vi "Define 1D Heat PDE BC (VIRef).vi"(0 "PDE in":refnum<class "NI_PDE.lvclass">, 1 "data":variant, 5 "Boundary Condition":refnum<vi>, 7 "type":T2 items=["Dirichlet", "Neumann"], 9 "position":T1 items=["Start X", "End X"], 11 "error in (no error)":errorcluster) -> (4 "PDE out":refnum<class "NI_PDE.lvclass">, 15 "error out":errorcluster)   [LabVIEW 2017, in "NI_PDE.lvlib"]
doc: "Defines the boundary condition of partial differential equations. You must manually select the polymorphic instance to use."
uses:
  <vilib>/gmath/NI_PDE.lvlib
  <vilib>/gmath/pde.llb/Common/PDE_BC Type.ctl
  <vilib>/gmath/pde.llb/PDEClass/NI_PDE.lvclass
  <vilib>/gmath/pde.llb/Common/PDE_BC Position 1D.ctl
  <vilib>/gmath/pde.llb/BCClass/BC_Evolut_1D_VIRef/NI_BC_Evolut_1D_VIRef.lvclass
  e:/builds/penguin/labview/branches/2017/dev/dist/vi.lib/gmath/pde.llb/BCClass/NI_BC.lvclass
  <vilib>/gmath/pde.llb/PDEClass/PDE_Heat_1D/NI_PDE_Heat_1D.lvclass
  e:/builds/penguin/labview/branches/2017/dev/dist/vi.lib/gmath/pde.llb/PDEClass/NI_PDE.lvclass
  <vilib>/gmath/pde.llb/BCClass/BC_Evolut_1D_VIRef/BC Data.ctl
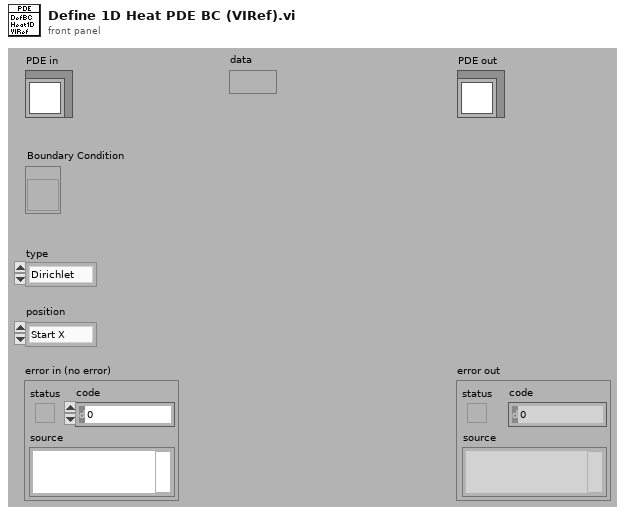
[diagram p1: front panel]
types:
  T1 = typedef "NI_PDE.lvlib/PDE_BC Position 1D.ctl" = i32
  T2 = typedef "NI_PDE.lvlib/PDE_BC Type.ctl" = i32
  T3 = typedef "NI_PDE.lvlib/NI_BC_Evolut_1D_VIRef.lvclass/BC Data.ctl" = cluster{"type":T2, "position":T1, "G":refnum<vi>, "data":variant}
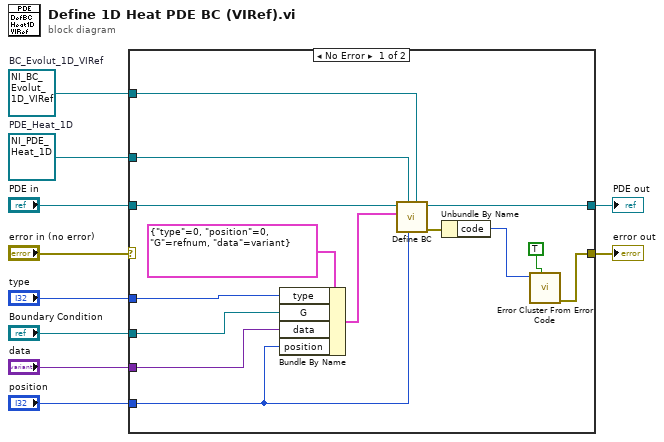
[diagram p0: block diagram]
diagram:
  w2 = refnum<class "NI_PDE_Heat_1D.lvclass"> refnum  # PDE_Heat_1D
  w1 = refnum<class "NI_BC_Evolut_1D_VIRef.lvclass"> refnum  # BC_Evolut_1D_VIRef
  n1 = case shown="No Error" "error in (no error)" {
    selector: "error in (no error)" -> [_ w26]
    tunnel: "PDE in" -> [w13 w25]
    tunnel: [w21 w25] -> w9
    tunnel: "position" -> [w15 _]
    tunnel: "data" -> [w16 _]
    tunnel: "Boundary Condition" -> [w17 _]
    tunnel: "type" -> [w18 _]
    tunnel: [w22 w26] -> w4
    tunnel: w2 -> [w12 _]
    tunnel: w1 -> [w11 _]
    frame No Error {
      n2 = Bundle By Name(cluster=T3 {"type"=0, "position"=0, "G"=refnum, "data"=variant} ("BC data"), "type"=w18, "G"=w17, "data"=w16, "position"=w15) -> (w14:T3)
      n3 = call <vilib>:"Define BC.vi"("target BC"=w11, "index"=w15, "target PDE"=w12, "BC"=w14, "PDE in"=w13) -> ("error out"=w20:errorcluster, "PDE out"=w21:refnum<class "NI_PDE.lvclass">)  [unwired: 2 in, 3 out]
      n4 = Unbundle By Name(w20) -> ("code"=w24:i32)
      n5 = call <vilib>:"Error Cluster From Error Code.vi"("show call chain? (False)"=TRUE, "error code (0)"=w24) -> ("error out"=w22:errorcluster)  [unwired: 1 in, 6 out]
    }
    frame Error {
    }
  }
  "PDE out" <- w9
  "error out" <- w4
